vi "read_Current_subvi.vi"(0 "Aardvark Handle":i32 min=0, 1 "Address (0x50)":u16=80 max=1023 format="%.0x", 3 "error in (no error)":errorcluster) -> (7 "Dup Aardvark Handle":i32, 9 "Current":dbl, 10 "error out":errorcluster)   [LabVIEW 2014]
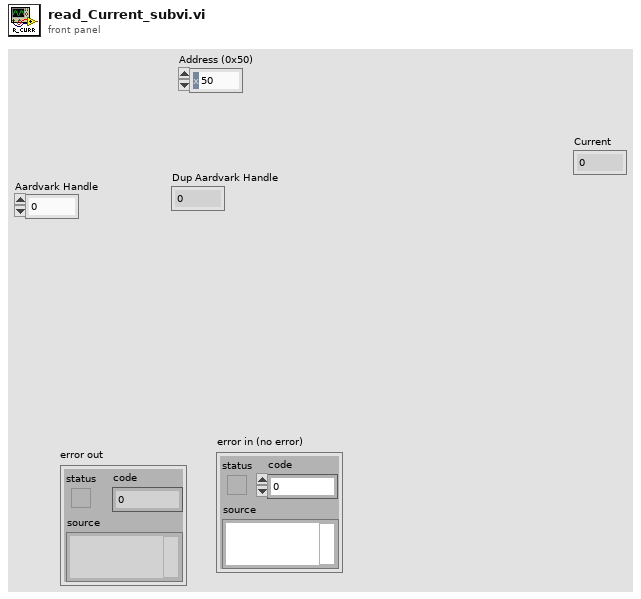
[diagram p1: front panel]
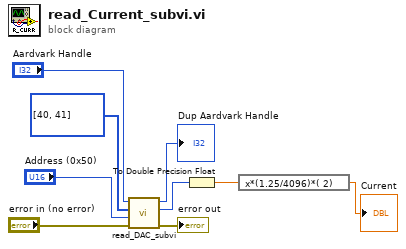
[diagram p0: block diagram]
diagram:
  n1 = call "read_DAC_subvi.vi"("error in (no error)"="error in (no error)", "Address (0x50)"="Address (0x50)", "DAC_ADD"=u16[] [40, 41], "Aardvark Handle"="Aardvark Handle") -> ("error out"=→"error out":errorcluster, "DAC Val"=w4:u16, "Dup Aardvark Handle"=→"Dup Aardvark Handle":i32)  [unwired: 3 in]
  n2 = To Double Precision Float(number=w4) -> (double precision float=w9:dbl)
  n3 = expression code="x*(1.25/4096)*( 2)"(w9) -> (→"Current":dbl)
